vi "Get value OUT1.vi"(0 "Keyence":T2={"Serial port sem"=refnum, "Serial port handle"="", "Baud rate"=9600}, 5 "error in":errorcluster) -> (11 "Start transfer":u32, 14 "Keyence out":T2={"Serial port sem"=refnum, "Serial port handle"="", "Baud rate"=9600}, 17 "Distance":dbl, 19 "error out":errorcluster)   [LabVIEW 2018]
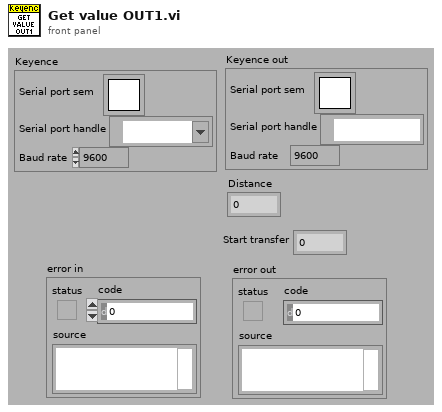
[diagram p1: front panel]
types:
  T1 = typedef "Semaphore RefNum" = refnum<k1>
  T2 = cluster{"Serial port sem":T1, "Serial port handle":refnum<visa-resource-name>, "Baud rate":u32}
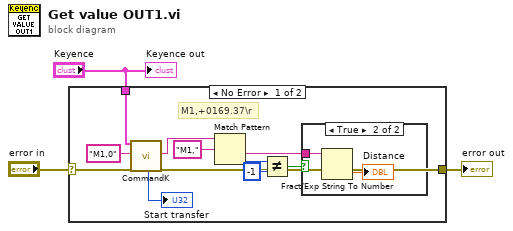
[diagram p0: block diagram]
diagram:
  n1 = case shown="No Error" "error in" {
    selector: "error in" -> [w14 w17]
    tunnel: [w7 w17] -> w3
    tunnel: "Keyence" -> [w6 _]
    frame No Error {
      # "M1,+0169.37\\r"
      n2 = call "CommandK.vi"("Keyence"=w6, "Command"="M1,0", "error in"=w14) -> ("Command time, ms"=→"Start transfer":u32, "Answer"=w4:string, "error out"=w7:errorcluster)  [unwired: 13 in, 1 out]
      n3 = Match Pattern(string=w4, regular expression="M1," ("string")) -> (after substring=w11:string, offset past match=w10:i32)  [unwired: 1 in, 2 out]
      n4 = Not Equal?(x=w10, y=-1) -> (x != y?=w8:bool)
      n5 = case shown="True" w8 {
        tunnel: w11 -> [_ w16]
        frame False {
        }
        frame True {
          n6 = Fract/Exp String To Number(string=w16) -> (number=→"Distance":dbl)  [unwired: 3 in, 1 out]
        }
      }
    }
    frame Error {
    }
  }
  "error out" <- w3
  "Keyence out" <- "Keyence"
